vi "Test App Error Handler is Configured Process Added before Start.vi"(8 "error in (no error)":errorcluster, 11 "Rig Test In":refnum<class "Application Test.lvclass">) -> (0 "error out":errorcluster, 3 "Rig Test Out":refnum<class "Application Test.lvclass">)   [LabVIEW 2020, in "Application Test.lvclass"]
uses:
  Application Test.lvclass
  C:/Program Files (x86)/National Instruments/LabVIEW 2020/vi.lib/Asteme/LUnit/Test Case.lvclass
  Mock Error Handler/Mock Error Handler.lvclass
  C:/Users/anton/Documents/GitHub/Triarc-Framework/source/Framework/Error Handler Interface/Error Handler Interface.lvclass
  Mock Process/Mock Process.lvclass
  C:/Users/anton/Documents/GitHub/Triarc-Framework/source/Framework/Process/Process.lvclass
  Framework/Process/Process.lvclass/Process.ctl
  Framework/Application/Application.lvclass/Application.ctl
  <vilib>/Asteme/LUnit/Test Case.lvclass/Test Case.ctl
  <vilib>/Asteme/LUnit/LUnit Assertion Result.lvclass/LUnit Assertion Result.ctl
  Framework/Application/Private/Add Process to Map.vi
  Framework/Process/Protected/Messaging/Enqueue Message.vi
  Framework/Process/Protected/SubVIs/Set Context.vi
  Framework/Process/Public/Lifecycle/Get Lifecycle State.vi
  <vilib>/Utility/error.llb/Clear Errors.vi
  Framework/Process/Protected/Messaging/Request Message.vi
  Framework/Process/Private/SubVIs/Wait for finish.vi
  Framework/Process/Private/SubVIs/Set Lifecycle State.vi
  <vilib>/Asteme/LUnit/Palette/Pass.vi
  <vilib>/Asteme/LUnit/Palette/Fail.vi
  <vilib>/Asteme/LUnit/Variant to string.vi
  <vilib>/Asteme/LUnit/Set Assertion Type.vi
  Framework/Process/Community/Leave Process Loop.vi
  Framework/Process/Private/SubVIs/Enqueue Request Message.vi
  <vilib>/Asteme/LUnit/Add test result.vi
  <vilib>/Asteme/LUnit/LUnit Write Passed.vi
  <vilib>/Asteme/LUnit/LUnit Get Test Case.vi
  <vilib>/Asteme/LUnit/Assertion Result/LUnit Get Test Name.vi
  <vilib>/Asteme/LUnit/LUnit Write Message.vi
  <vilib>/Asteme/LUnit/LUnit Write Description.vi
  <vilib>/Asteme/LUnit/LUnit Write Assertion Type.vi
  <vilib>/Asteme/LUnit/Read Test Case Name.vi
  Framework/Application/Application.lvclass
  <vilib>/Utility/error.llb/Error Cluster From Error Code.vi
  Framework/Application/Private/Update Context for Owned Processes.vi
  Framework/Process/Private/SubVIs/Wait for Response Message.vi
  <vilib>/Utility/Data Type/Get Type Information.vi
  <vilib>/Utility/LVClass/Get LV Class Name.vi
  Framework/Process/Process.lvclass
  <vilib>/Asteme/LUnit/LUnit Assertion Result.lvclass
  <vilib>/Asteme/LUnit/Test Case.lvclass
  Support/Framework Test Support.lvlib
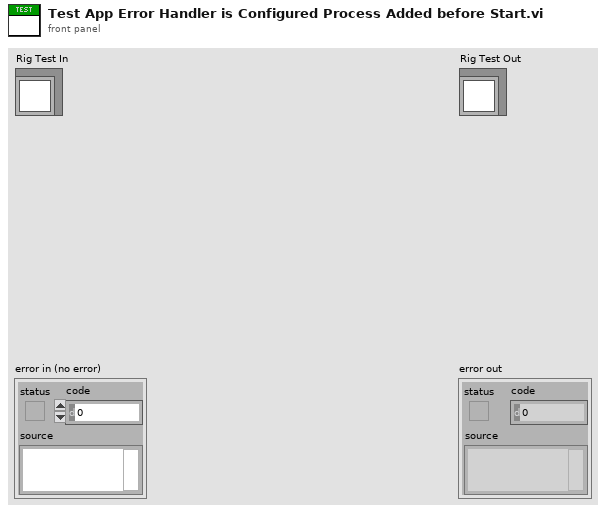
[diagram p1: front panel]
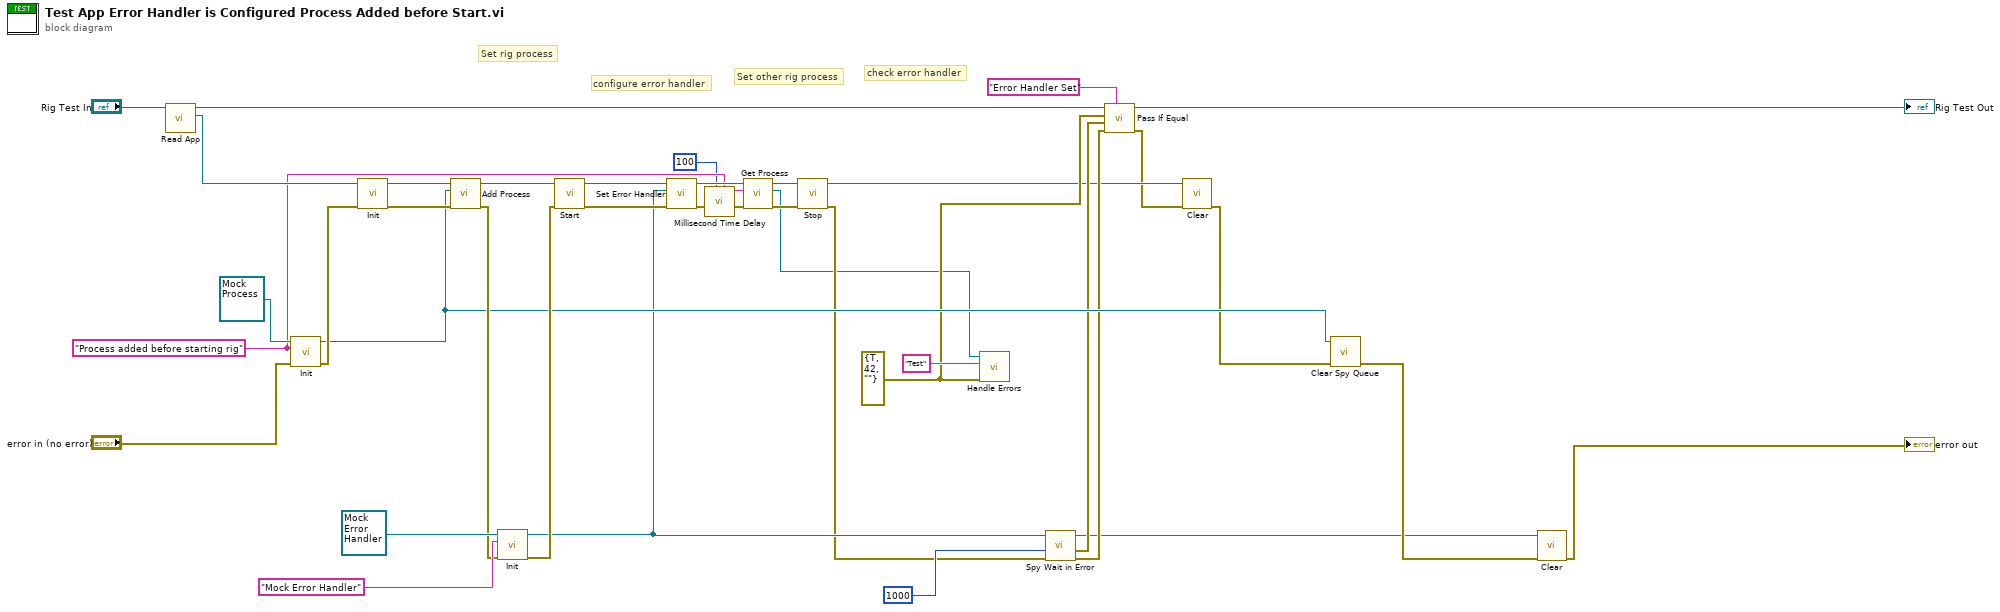
[diagram p0: block diagram]
diagram:
  w18 = errorcluster {"status"=TRUE, "code"=42, "source"=""} ("error in (no error)")
  w5 = "Process added before starting rig" ("Name")
  # "check error handler"
  # "Set other rig process"
  # "configure error handler"
  # "Set rig process"
  n1 = call "Read App.vi"("Application Test In"="Rig Test In") -> ("App out"=w38:refnum<class "Application.lvclass">, "Application Test Out"=w13:refnum<class "Application Test.lvclass">)  [unwired: 8 in, 1 out]
  n2 = call-dynamic "Init.vi"("error in (no error)"="error in (no error)", "Name"=w5, "Mock Process In"=refnum<class "Mock Process.lvclass"> refnum ("Mock Process.lvclass")) -> ("error out"=w28:errorcluster, "Mock Process Out"=w23:refnum<class "Mock Process.lvclass">)  [unwired: 7 in]
  n3 = call-dynamic "Init.vi"("error in (no error)"=w28, "Process In"=w38) -> ("error out"=w26:errorcluster, "Process Out"=w37:refnum<class "Application.lvclass">)  [unwired: 8 in]
  n4 = call "Add Process.vi"("error in (no error)"=w26, "Process"=w23, "Rig In"=w37) -> ("error out"=w25:errorcluster, "Rig Out"=w27:refnum<class "Application.lvclass">)  [unwired: 7 in]
  n5 = call-dynamic "Init.vi"("error in (no error)"=w25, "Name"="Mock Error Handler", "Mock Error Handler In"=refnum<class "Mock Error Handler.lvclass"> refnum ("Mock Error Handler.lvclass")) -> ("error out"=w31:errorcluster, "Mock Error Handler Out"=w10:refnum<class "Mock Error Handler.lvclass">)  [unwired: 7 in]
  n6 = call "Start.vi"("error in (no error)"=w31, "Process In"=w27) -> ("error out"=w24:errorcluster, "Process Out"=w36:refnum<class "Application.lvclass">)  [unwired: 8 in]
  n7 = call "Set Error Handler.vi"("error in (no error)"=w24, "Error Handler"=w10, "Process In"=w36) -> ("error out"=w35:errorcluster, "Process Out"=w7:refnum<class "Application.lvclass">)  [unwired: 7 in]
  n8 = call "Millisecond Time Delay.vi"("milliseconds to wait"=u32 100, "error in (no error)"=w35) -> ("error out"=w2:errorcluster)  [unwired: 7 in]
  n9 = call "Get Process.vi"("error in (no error)"=w2, "Process Name"=w5, "Rig In"=w7) -> ("error out"=w8:errorcluster, "App Process"=w3:refnum<class "Process.lvclass">, "Rig Out"=w6:refnum<class "Application.lvclass">)  [unwired: 6 in]
  n10 = call "Stop.vi"("error in (no error)"=w8, "Process In"=w6) -> ("error out"=w4:errorcluster, "Process Out"=w14:refnum<class "Application.lvclass">)  [unwired: 7 in, 1 out]
  n11 = call-dynamic "Handle Errors.vi"("error in (no error)"=w18, "Location"="Test", "Process In"=w3) -> ()  [unwired: 7 in, 2 out]
  n12 = call "Spy Wait in Error.vi"("error in (no error)"=w4, "timeout in ms (-1)"=1000, "Mock Error Handler In"=w10) -> ("error out"=w16:errorcluster, "Errors"=w17:errorcluster, "Mock Error Handler Out"=w9:refnum<class "Mock Error Handler.lvclass">)  [unwired: 4 in, 2 out]
  n13 = call <vilib>:"Pass If Equal.vi"("Description"="Error Handler Set", "error in (no error)"=w16, "Actual"=w17, "Expected"=w18, "Test Case In"=w13) -> ("error out"=w11:errorcluster, "Test Case Out"=→"Rig Test Out":refnum<class "Application Test.lvclass">)  [unwired: 5 in]
  n14 = call-dynamic "Clear.vi"("error in (no error)"=w11, "Application In"=w14) -> ("error out"=w22:errorcluster)  [unwired: 8 in, 1 out]
  n15 = call-dynamic "Clear Spy Queue.vi"("error in (no error)"=w22, "Mock Process In"=w23) -> ("error out"=w21:errorcluster)  [unwired: 8 in, 1 out]
  n16 = call-dynamic "Clear.vi"("error in (no error)"=w21, "Mock Process In"=w9) -> ("error out"=→"error out":errorcluster)  [unwired: 8 in, 1 out]
